vi "Degrees to Radians (Array DBL).vi"(3 "angles (deg)":dbl[](array[numeric])) -> (1 "angles (rad)":dbl[](array[numeric]))   [LabVIEW 2020, in "NI_AngleManipulation.lvlib"]
doc: "Converts a 1D array of angles from degrees to radians."
uses:
  <vilib>/Utility/AngleManip/NI_AngleManipulation.lvlib
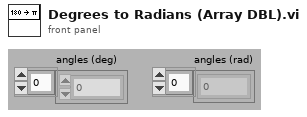
[diagram p1: front panel]
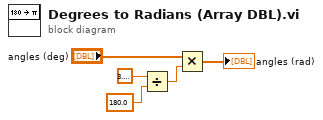
[diagram p0: block diagram]
diagram:
  n1 = Divide(x=3.141592653589793, y=180.0) -> (x/y=w3:dbl)
  n2 = Multiply(x="angles (deg)", y=w3) -> (x*y=→"angles (rad)":dbl[])
